vi "Tusk.SendMessage.vi"(5 "Priority?":bool, 7 "Timeout (ms)(-1)":i32=-1, 8 "error in (no error)":errorcluster, 9 "Data":variant, 10 "Local Tusk.Message / Global Tusk.Local Tusk. Message":string, 11 "Tusk in":refnum<class "Tusk.lvclass">) -> (0 "error out":errorcluster, 3 "Tusk out":refnum<class "Tusk.lvclass">)   [LabVIEW 2018, in "Application.lvlib" / "Tusk.lvclass"]
uses:
  Tusk.lvclass
  Tusk.lvclass/Tusk.ctl
  Message Class/Message.lvclass/Message.ctl
  Dictionary Class/Dictionary.lvclass/Dictionary.ctl
  Exceptions Class/VIs/Invalid Type.vi
  Tusk.GetTuskFromDictionary.vi/3fa77438-33e4-48e7-a501-c74b9750b9f8.vi
  Tusk.GetDictionary.vi
  Tusk.GetTuskFromDictionary.vi/bb4b4b2f-5120-4767-9776-c61ed956de36.vi
  Dictionary Class/VIs/Get Data DVR.vi
  <vilib>/Utility/error.llb/Trim Whitespace.vi
  Message Class/Message.lvclass
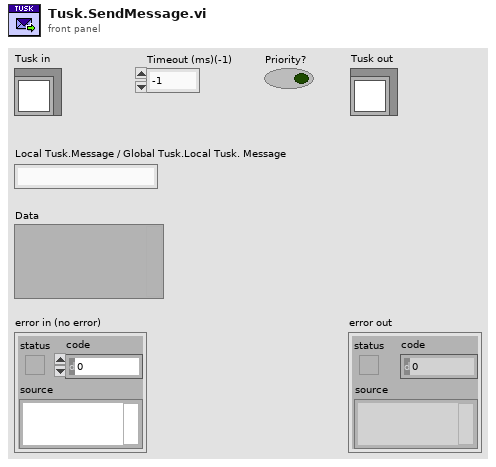
[diagram p1: front panel]
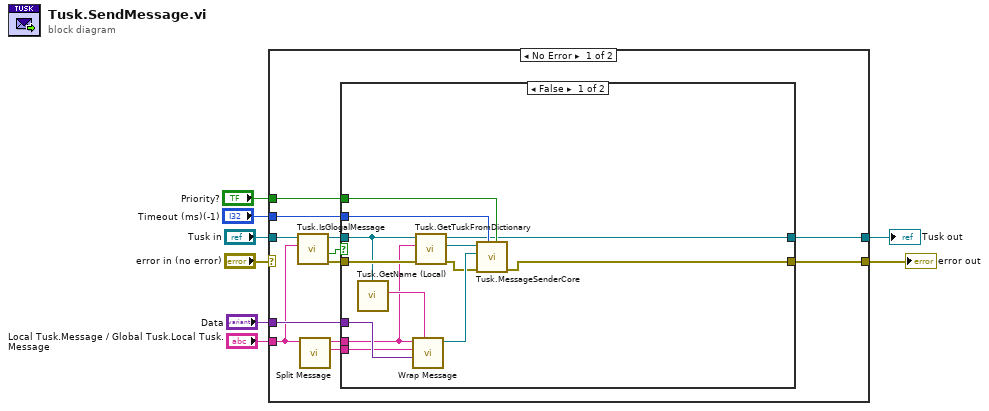
[diagram p0: block diagram]
diagram:
  n1 = case shown="No Error" "error in (no error)" {
    selector: "error in (no error)" -> [_ w37]
    tunnel: [w10 w37] -> w7
    tunnel: [w9 w36] -> w5
    tunnel: "Tusk in" -> [w20 w36]
    tunnel: "Local Tusk.Message / Global Tusk.Local Tusk. Message" -> [w13 _]
    tunnel: "Data" -> [w14 _]
    tunnel: "Priority?" -> [w12 _]
    tunnel: "Timeout (ms)(-1)" -> [w11 _]
    frame No Error {
      n2 = call "Tusk.IsGlogalMessage.vi"("Message"=w13, "Tusk in"=w20) -> ("error out"=w19:errorcluster, "Is Global Tusk Message?"=w18:bool, "Tusk out"=w17:refnum<class "Tusk.lvclass">)  [unwired: 7 in]
      n3 = call "Split Message.vi"("Recipient.Message"=w13) -> ("Message"=w16:string, "Recipient"=w15:string)  [unwired: 8 in, 1 out]
      n4 = case shown="False" w18 {
        tunnel: w19 -> [w26 w34]
        tunnel: w17 -> [w25 w35]
        tunnel: w16 -> [w32 _]
        tunnel: w15 -> [w21 _]
        tunnel: w14 -> [w33 _]
        tunnel: [w24 w35] -> w9
        tunnel: w12 -> [w30 _]
        tunnel: w11 -> [w31 _]
        tunnel: [w29 w34] -> w10
        frame False {
          n5 = call "Tusk.GetName (Local).vi"("Tusk in"=w25) -> ("Name(Local)"=w28:string)  [unwired: 8 in, 2 out]
          n6 = call "Wrap Message.vi"("Sender"=w28, "Data"=w33, "Message"=w32, "Recipient"=w21) -> ("Message out"=w27:refnum<class "Message.lvclass">)  [unwired: 6 in, 1 out]
          n7 = call "Tusk.GetTuskFromDictionary.vi"("error in (no error)"=w26, "Name (Local)"=w21, "Tusk in"=w25) -> ("error out"=w23:errorcluster, "Tusk"=w22:refnum<class "Tusk.lvclass">, "Tusk out"=w24:refnum<class "Tusk.lvclass">)  [unwired: 6 in]
          n8 = call "Tusk.MessageSenderCore.vi"("Priority?"=w30, "Timeout (ms)(-1)"=w31, "error in (no error)"=w23, "Message"=w27, "Tusk in"=w22) -> ("error out"=w29:errorcluster)  [unwired: 4 in, 2 out]
        }
        frame True {
          # "#ToDo work on global message sender"
        }
      }
    }
    frame Error {
    }
  }
  "error out" <- w7
  "Tusk out" <- w5
